vi "Linear Fit.vi"(0 "Y":dbl[](array[numeric]), 5 "X":dbl[](array[numeric]), 7 "Weight":dbl[](array[numeric]), 9 "tolerance":dbl=0.0001 format="%#_3g", 11 "method":T2 items=["Least Square", "Least Absolute Residual", "Bisquare"], 12 "parameter bounds":T1={"slope min"=-inf, "slope max"=inf, "intercept min"=-inf, "intercept max"=inf}) -> (4 "Best Linear Fit":dbl[](array[numeric]), 6 "slope":dbl, 8 "intercept":dbl, 14 "residue":dbl, 15 "error":i32)   [LabVIEW 2014, in "NI_AALPro.lvlib"]
doc: "Returns the linear fit of a data set (<B>X</B>, <B>Y</B>) using the Least Square, Least Absolute Residual, or Bisquare method."
uses:
  NI_AALPro.lvlib
  Curve Fitting Criteria.ctl
  lvanlys.dll
panel:
  # "Constrained Linear Fit"
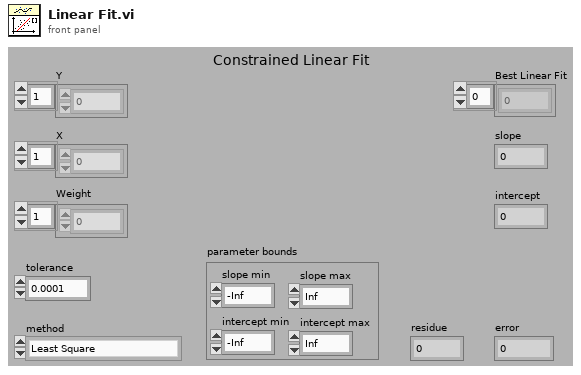
[diagram p1: front panel]
types:
  T1 = cluster{"slope min":dbl, "slope max":dbl, "intercept min":dbl, "intercept max":dbl}
  T2 = typedef "NI_AALPro.lvlib/Curve Fitting Criteria.ctl" = u16
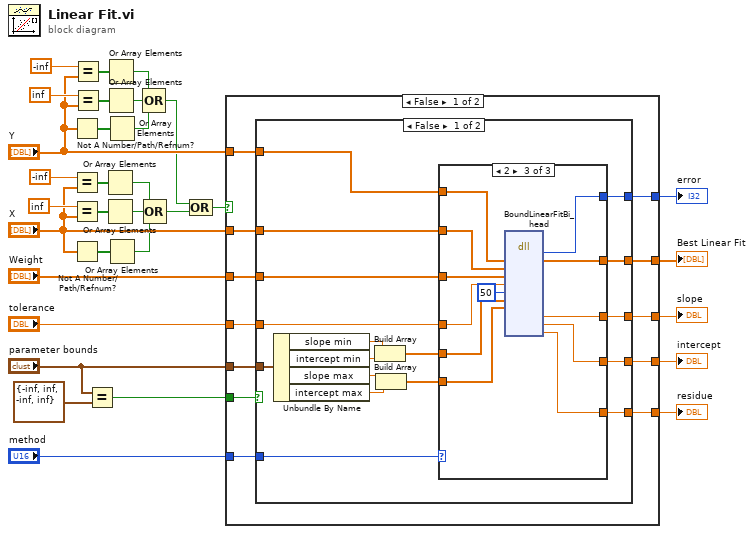
[diagram p0: block diagram]
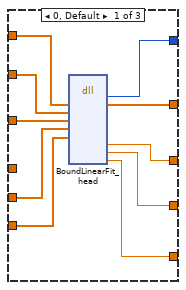
[diagram p2: hidden frame]
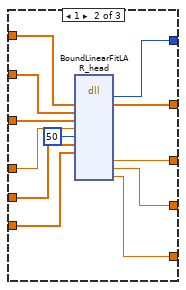
[diagram p3: hidden frame]
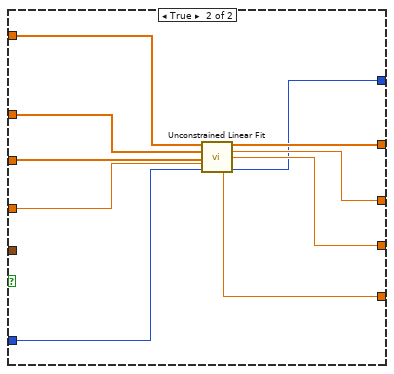
[diagram p4: hidden frame]
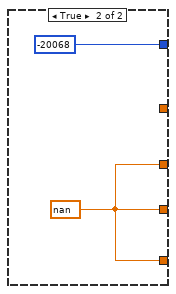
[diagram p5: hidden frame]
diagram:
  n1 = Not A Number/Path/Refnum?(number/path/refnum="Y") -> (NaN/Path/Refnum?=w21:bool[])
  n2 = Equal?(x=-inf, y="X") -> (x = y?=w10:bool[])
  n3 = Equal?(x=inf, y="X") -> (x = y?=w9:bool[])
  n4 = Not A Number/Path/Refnum?(number/path/refnum="X") -> (NaN/Path/Refnum?=w20:bool[])
  n5 = Equal?(x=-inf, y="Y") -> (x = y?=w14:bool[])
  n6 = Equal?(x=inf, y="Y") -> (x = y?=w15:bool[])
  n7 = Equal?(x="parameter bounds", y=T1 {"slope min"=-inf, "slope max"=inf, "intercept min"=-inf, "intercept max"=inf} ("parameter bounds 2")) -> (x = y?=w23:bool)
  n8 = Or Array Elements(Boolean array=w10) -> (logical OR=w4:bool)
  n9 = Or Array Elements(Boolean array=w9) -> (logical OR=w5:bool)
  n10 = Or Array Elements(Boolean array=w14) -> (logical OR=w12:bool)
  n11 = Or Array Elements(Boolean array=w15) -> (logical OR=w13:bool)
  n12 = Or Array Elements(Boolean array=w21) -> (logical OR=w11:bool)
  n13 = Or Array Elements(Boolean array=w20) -> (logical OR=w3:bool)
  n14 = Compound Arithmetic op=OR(w12, w13, w11) -> (w1:bool)
  n15 = Compound Arithmetic op=OR(w4, w5, w3) -> (w2:bool)
  n16 = Compound Arithmetic op=OR(w1, w2) -> (w19:bool)
  n17 = case shown="False" w19 {
    tunnel: "tolerance" -> [w44 _]
    tunnel: [w43 _] -> w31
    tunnel: [w42 w106] -> w30
    tunnel: [w41 w106] -> w29
    tunnel: [w40 w106] -> w28
    tunnel: [w39 -20068 ("error")] -> w27
    tunnel: "method" -> [w38 _]
    tunnel: "parameter bounds" -> [w37 _]
    tunnel: w23 -> [w36 _]
    tunnel: "Y" -> [w35 _]
    tunnel: "X" -> [w34 _]
    tunnel: "Weight" -> [w33 _]
    frame False {
      n18 = case shown="False" w36 {
        tunnel: w35 -> [w61 w105]
        tunnel: w34 -> [w60 w103]
        tunnel: w33 -> [w59 w102]
        tunnel: w44 -> [w58 w101]
        tunnel: [w57 w104] -> w43
        tunnel: [w56 w99] -> w42
        tunnel: [w55 w98] -> w41
        tunnel: [w54 w96] -> w40
        tunnel: [w53 w97] -> w39
        tunnel: w38 -> [w52 w100]
        tunnel: w37 -> [w51 _]
        frame False {
          n19 = Unbundle By Name(w51) -> ("slope min"=w50:dbl, "intercept min"=w49:dbl, "slope max"=w48:dbl, "intercept max"=w47:dbl)
          n20 = Build Array(w50, w49) -> (w46:dbl[])
          n21 = Build Array(w48, w47) -> (w45:dbl[])
          n22 = case shown="2" w52 {
            tunnel: w61 -> [w71 w83 w95]
            tunnel: w60 -> [w70 w82 w94]
            tunnel: w59 -> [w69 w81 w93]
            tunnel: w58 -> [_ w80 w92]
            tunnel: [w68 w78 w90] -> w57
            tunnel: [w67 w77 w89] -> w56
            tunnel: [w66 w76 w88] -> w55
            tunnel: [w65 w75 w87] -> w54
            tunnel: [w64 w74 w86] -> w53
            tunnel: w46 -> [w63 w73 w85]
            tunnel: w45 -> [w62 w72 w84]
            frame 0, Default {
              n23 = dll-call lib="C:/Program Files (x86)/National Instruments/LabVIEW 2014/resource/lvanlys.*" fn="BoundLinearFit_head"("y"=w71, "x"=w70, "weight"=w69, "minBound"=w63, "maxBound"=w62) -> ("return type"=w64:i32, "y"=w68:dbl[], "slope"=w67:dbl, "intercept"=w66:dbl, "mse"=w65:dbl)  [unwired: 7 in, 5 out]
            }
            frame 1 {
              n24 = dll-call lib="C:/Program Files (x86)/National Instruments/LabVIEW 2014/resource/lvanlys.*" fn="BoundLinearFitLAR_head"("y"=w83, "x"=w82, "weight"=w81, "tolerance"=w80, "maxIter"=50, "minBound"=w73, "maxBound"=w72) -> ("return type"=w74:i32, "y"=w78:dbl[], "slope"=w77:dbl, "intercept"=w76:dbl, "meanErr"=w75:dbl)  [unwired: 8 in, 6 out]
            }
            frame 2 {
              n25 = dll-call lib="C:/Program Files (x86)/National Instruments/LabVIEW 2014/resource/lvanlys.*" fn="BoundLinearFitBi_head"("y"=w95, "x"=w94, "weight"=w93, "tolerance"=w92, "maxIter"=50, "minBound"=w85, "maxBound"=w84) -> ("return type"=w86:i32, "y"=w90:dbl[], "slope"=w89:dbl, "intercept"=w88:dbl, "mse"=w87:dbl)  [unwired: 8 in, 6 out]
            }
          }
        }
        frame True {
          n26 = call "Unconstrained Linear Fit.vi"("Y"=w105, "X"=w103, "Weight"=w102, "tolerance"=w101, "method"=w100) -> ("Best Linear Fit"=w104:dbl[], "slope"=w99:dbl, "intercept"=w98:dbl, "residue"=w96:dbl, "error"=w97:i32)  [unwired: 6 out]
        }
      }
    }
    frame True {
      w106 = nan ("slope")
    }
  }
  "intercept" <- w29
  "slope" <- w30
  "Best Linear Fit" <- w31
  "error" <- w27
  "residue" <- w28
